vi "TriggerFunction.vi"(10 "Input Cluster":T1={"Threshold"=0.0, "Waveform"={"t0"=timestamp(0 s since 1904-01-01), "dt"=1.0, "Y"=[]}, "hysteresis"=0.0, "location mode"=0, "error in (no error)"={"status"=FALSE, "code"=0, "source"=""}, "trigger slope"=1} {"trigger slope" items=["Falling Edge", "Rising Edge"]; "location mode" items=["Index", "Time"]; "hysteresis" format="%.2p"}) -> (0 "error out":errorcluster, 1 "trigger detected?":bool, 3 "Trigger Locations":i32[](array[numeric]))   [LabVIEW 2014]
uses:
  <vilib>/measure/mamon.llb/Trigger Detection for 1 Channel.vi
  <vilib>/measure/NI_MAPro.lvlib
panel:
  # "Inputs"
  # "Outputs"
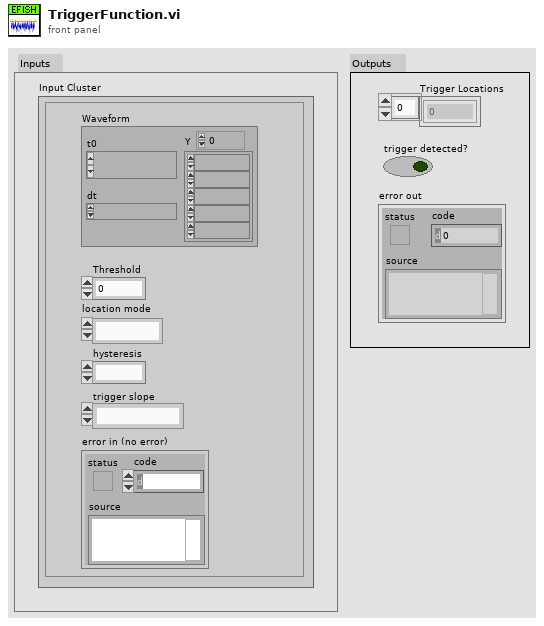
[diagram p1: front panel]
types:
  T1 = cluster{"Threshold":dbl, "Waveform":waveform(dbl), "hysteresis":dbl, "location mode":u16, "error in (no error)":errorcluster, "trigger slope":u16}
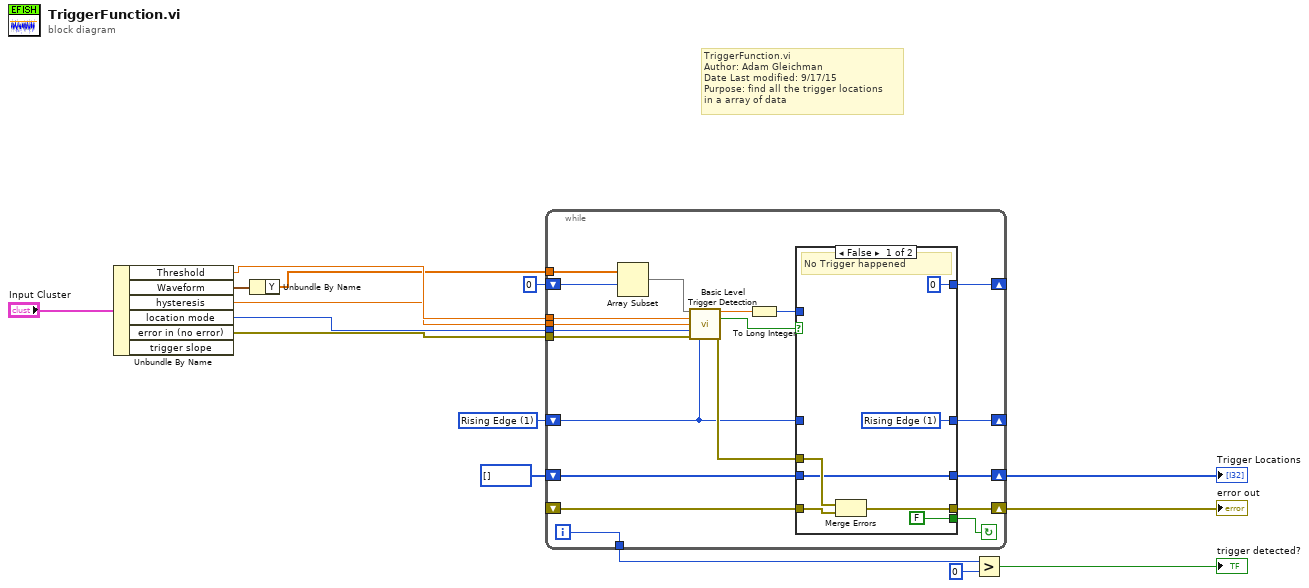
[diagram p0: block diagram]
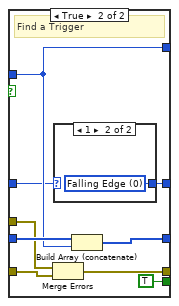
[diagram p2: hidden frame]
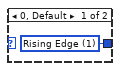
[diagram p3: hidden frame]
diagram:
  w9 = u16 1 items=["Falling Edge", "Rising Edge"] ("trigger slope")
  # "TriggerFunction.vi\nAuthor: Adam Gleichman\nDate Last modified: 9/17/15\nPurpose: find all the trigger locations\nin a array of data"
  n1 = Unbundle By Name("Input Cluster") -> ("Threshold"=w13:dbl, "Waveform"=w14:waveform(dbl), "hysteresis"=w12:dbl, "location mode"=w11:u16, "error in (no error)"=w10:errorcluster)  [unwired: 1 out]
  n2 = Unbundle By Name(w14) -> ("Y"=w8:dbl[])
  n3 = while {
    tunnel: w13 -> [w35]
    tunnel: w12 -> [w34]
    tunnel: w11 -> [w33]
    tunnel: w10 -> [w32]
    tunnel: w8 -> [w26]
    shift-right: [w27] -> _
    shift-left: 0 ("trigger location") -> [w25]
    shift-right: [w21] -> w1
    shift-left: i32[] [] -> [w22]
    shift-right: [w20] -> _
    shift-left: w9 -> [w19]
    tunnel: [w18] -> w5
    shift-right: [w16] -> w2
    shift-left: _ -> [w17]
    i -> [w18]
    stop <- w30 continue-if-true
    n4 = Array Subset(array=w26, index=w25) -> (w23:dbl[])  [unwired: 1 in]
    n5 = call-poly <vilib>:"Basic Level Trigger Detection.vi"("signal in"=w23, "level"=w35, "hysteresis"=w34, "location mode"=w33, "error in (no error)"=w32, "trigger slope"=w19) -> ("trigger location"=w29:dbl, "trigger detected?"=w31:bool, "error out"=w28:errorcluster)  [unwired: 7 in]
    n6 = To Long Integer(number=w29) -> (32bit integer=w24:i32)
    n7 = case shown="False" w31 {
      tunnel: [FALSE TRUE] -> w30
      tunnel: w24 -> [_ w49]
      tunnel: w28 -> [w39 w45]
      tunnel: [0 w49] -> w27
      tunnel: w22 -> [w36 w50]
      tunnel: [w36 w48] -> w21
      tunnel: [w40 w46] -> w20
      tunnel: w19 -> [_ w47]
      tunnel: w17 -> [w37 w44]
      tunnel: [w38 w43] -> w16
      frame False {
        w40 = u16 1 items=["Falling Edge", "Rising Edge"] ("trigger slope")
        # "No Trigger happened"
        n8 = Merge Errors(w39, w37) -> (w38:errorcluster)
      }
      frame True {
        # "Find a Trigger"
        n9 = Merge Errors(w45, w44) -> (w43:errorcluster)
        n10 = case shown="1" w47 {
          tunnel: [w52 w53] -> w46
          frame 0, Default {
            w52 = u16 1 items=["Falling Edge", "Rising Edge"] ("trigger slope")
          }
          frame 1 {
            w53 = u16 0 items=["Falling Edge", "Rising Edge"] ("trigger slope")
          }
        }
        n11 = Build Array (concatenate)(w50, w49) -> (w48:i32[])
      }
    }
  }
  "error out" <- w2
  "Trigger Locations" <- w1
  n12 = Greater?(x=w5, y=0) -> (0:→"trigger detected?":bool)
